vi "Camera_Config.vi"(5 "Crop?":bool, 6 "Camera":T5, 7 "error in":errorcluster, 8 "input cluster":T1={"L16 Linear Actuator"="", "XE 1000 Pump"="", "Camera1"="", "Camera2"="", "Camera1_IMG"=refnum, "Camera2_IMG"=refnum, "Img_Capt"=FALSE, "Actuator"=FALSE, "Pump"=FALSE, "Cam 1"=FALSE, "Cam 2"=FALSE, "Empty_Refill"=FALSE, "Crop"=FALSE, "Light intensity"=100, "Exposure Time"=1000.0, "Sample Name"="Test Sample", "Operator"="MRJ", "Calibration 1"=path "C:/Users/au540322/Desktop/IHS_Project/images/Debris/Debris_0/Debris_0_2019_06_01-23-32-49-686.PNG", "Calibration 2"=path "C:/Users/au540322/Desktop/IHS_Project/images/Debris/Debris_0/Debris_0_2019_06_01-23-32-49-686.PNG", "Framerate"=1, "Timeout Sample"=0, "Collection date"="MRJ", "Sample size threshold"=1, "Empty start"=1, "Command"="MRJ", "Calibration Image 1"=refnum, "Calibration Image 2"=refnum, "Original Image 1"=refnum, "Original Image 2"=refnum, "Processing Image 1"=refnum, "Processing Image 2"=refnum, "Object Image 1"=refnum, "Object Image 2"=refnum, "Cam 1 - save queue"=refnum, "Cam 2 - save queue"=refnum, "Station"="", "Species Name"="", "Other Notes"="", "Aperture"=enum."Item 0", "Image Process Queue Size"=500, "Image Save Queue Size"=500, "Overload threshold"=500, "Max Framerate"=100, "Blue Plane Image"=refnum, "Subtract Image"=refnum, "Binary Image 1"=refnum, "ROI mask allocation"=refnum, "Rectangle 1"={"Left"=0, "Top"=0, "Right"=0, "Bottom"=0, "Rotation"=0.0}, "Rectangle 2"={"Left"=0, "Top"=0, "Right"=0, "Bottom"=0, "Rotation"=0.0}, "Binary Image 2"=refnum, "Detection Region %"=0.0, "Cam 1 queue"=refnum, "Cam 2 queue"=refnum, "Detect image 1"=refnum, "Detect image 2"=refnum, "Detect 1"=path "C:/Users/au540322/Desktop/IHS_Project/images/Debris/Debris_0/Debris_0_2019_06_01-23-32-49-686.PNG", "Detect 2"=path "C:/Users/au540322/Desktop/IHS_Project/images/Debris/Debris_0/Debris_0_2019_06_01-23-32-49-686.PNG", "Max large object threshold"=0, "Open(T)/Close(F)"=FALSE} {"Rectangle 2"."Rotation" format="%.2f"; "Rectangle 2"."Left" scale=0.0..1024.0; "Rectangle 2"."Right" scale=0.0..1024.0; "Rectangle 1"."Rotation" format="%.2f"; "Rectangle 1"."Left" scale=0.0..1024.0; "Rectangle 1"."Right" scale=0.0..1024.0; "Max Framerate" min=1; "Overload threshold" min=1; "Image Save Queue Size" min=1; "Image Process Queue Size" min=1; "Empty start" min=1; "Sample size threshold" min=1; "Framerate" min=1; "Light intensity" scale=0.0..100.0}, 9 "Detect Movement":bool, 10 "Refnum in":T2="cam2") -> (0 "error out":errorcluster, 3 "Refnum out":T2="cam2")   [LabVIEW 2019]
doc: "Configures basler cameras for image acquisition with cropped aspectratio."
uses:
  <vilib>/userdefined/High Color/IMAQdx.ctl
  Camera_ID.ctl
  controls/Data.ctl
  <vilib>/vision/Image Controls.llb/IMAQ Image.ctl
  <resource>/objmgr/imaqdx.rc
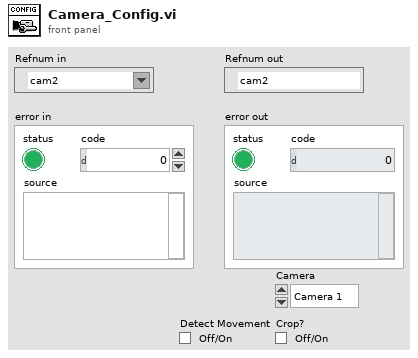
[diagram p1: front panel]
types:
  T1 = typedef "Data.ctl" = cluster{"L16 Linear Actuator":refnum<visa-resource-name>, "XE 1000 Pump":refnum<visa-resource-name>, "Camera1":T2, "Camera2":T2, "Camera1_IMG":T3, "Camera2_IMG":T3, "Img_Capt":bool, "Actuator":bool, "Pump":bool, "Cam 1":bool, "Cam 2":bool, "Empty_Refill":bool, "Crop":bool, "Light intensity":i32, "Exposure Time":dbl, "Sample Name":string, "Operator":string, "Calibration 1":path, "Calibration 2":path, "Framerate":i32, "Timeout Sample":i32, "Collection date":string, "Sample size threshold":i32, "Empty start":u32, "Command":string, "Calibration Image 1":T3, "Calibration Image 2":T3, "Original Image 1":T3, "Original Image 2":T3, "Processing Image 1":T3, "Processing Image 2":T3, "Object Image 1":T3, "Object Image 2":T3, "Cam 1 - save queue":refnum<queue>, "Cam 2 - save queue":refnum<queue>, "Station":string, "Species Name":string, "Other Notes":string, "Aperture":enum32{"Item 0", "Item 1", "Item 2", "Item 3"}, "Image Process Queue Size":i32, "Image Save Queue Size":i32, "Overload threshold":i32, "Max Framerate":i32, "Blue Plane Image":T3, "Subtract Image":T3, "Binary Image 1":T3, "ROI mask allocation":T3, "Rectangle 1":T4, "Rectangle 2":T4, "Binary Image 2":T3, "Detection Region %":dbl, "Cam 1 queue":refnum<queue>, "Cam 2 queue":refnum<queue>, "Detect image 1":T3, "Detect image 2":T3, "Detect 1":path, "Detect 2":path, "Max large object threshold":i32, "Open(T)/Close(F)":bool}
  T2 = typedef "IMAQdx.ctl" = refnum<k21>
  T3 = typedef "IMAQ Image.ctl" = refnum<image>
  T4 = typedef "IMAQ Rectangle" = cluster{"Left":i32, "Top":i32, "Right":i32, "Bottom":i32, "Rotation":dbl}
  T5 = typedef "Camera_ID.ctl" = enum16{"Camera 1", "Camera 2"}
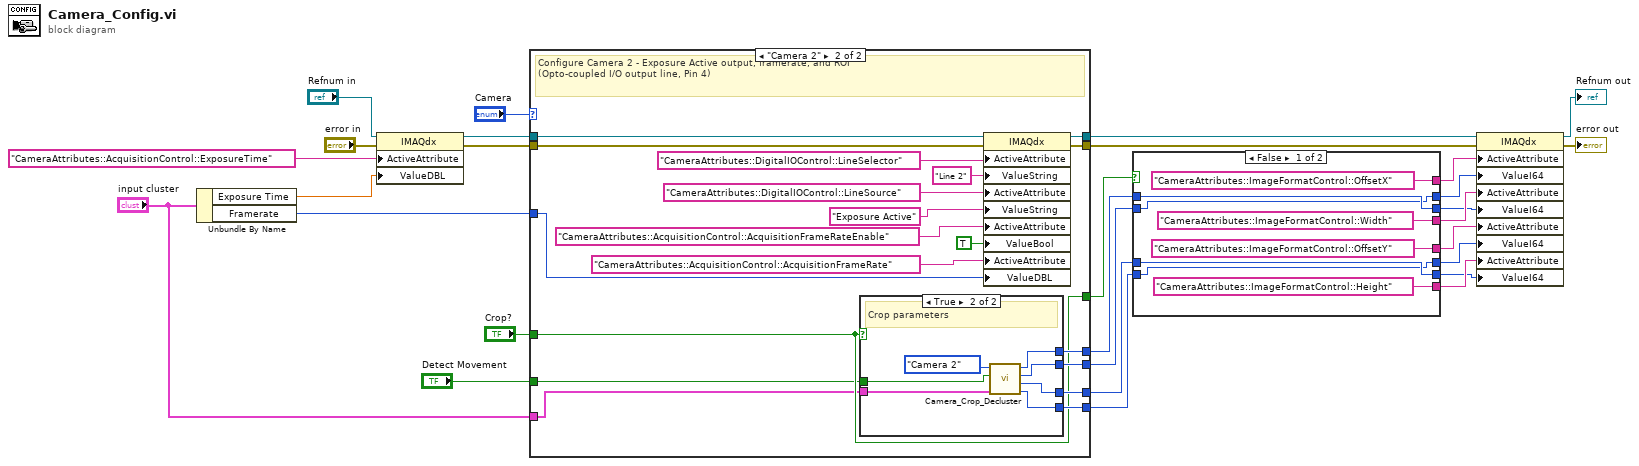
[diagram p0: block diagram]
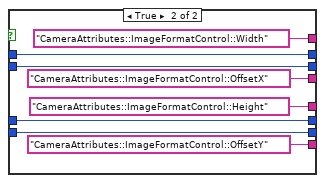
[diagram p2: hidden frame]
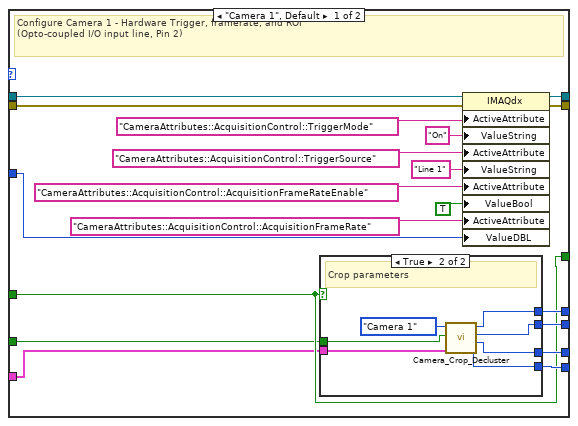
[diagram p3: hidden frame]
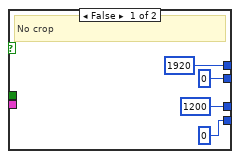
[diagram p4: hidden frame]
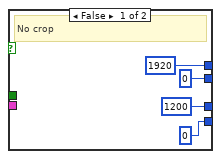
[diagram p5: hidden frame]
diagram:
  n1 = Unbundle By Name("input cluster") -> ("Exposure Time"=w23:dbl, "Framerate"=w22:i32)
  n2 = property class="IMAQdx"(reference="Refnum in", error in="error in", "ActiveAttribute"="CameraAttributes::AcquisitionControl::ExposureTime", "ValueDBL"=w23) -> (reference out=w14:T2, error out=w25:errorcluster)
  n3 = case shown="\"Camera 2\"" "Camera" {
    tunnel: w14 -> [w47 w76]
    tunnel: [w46 w74] -> w12
    tunnel: w25 -> [w45 w75]
    tunnel: [w44 w73] -> w21
    tunnel: w22 -> [w36 w66]
    tunnel: [w34 w65] -> w6
    tunnel: [w35 w64] -> w9
    tunnel: [w32 w62] -> w4
    tunnel: [w33 w63] -> w8
    tunnel: "Crop?" -> [w31 w61]
    tunnel: [w31 w61] -> w11
    tunnel: "input cluster" -> [w30 w60]
    tunnel: "Detect Movement" -> [w29 w59]
    frame "Camera 1", Default {
      # "Configure Camera 1 - Hardware Trigger, framerate, and ROI \n(Opto-coupled I/O input line, Pin 2)"
      n4 = case shown="True" w31 {
        tunnel: [i64 1920 w57] -> w35
        tunnel: [1200 w55] -> w34
        tunnel: [i64 0 w56] -> w33
        tunnel: [0 w54] -> w32
        tunnel: w30 -> [_ w53]
        tunnel: w29 -> [_ w52]
        frame False {
          # "No crop"
        }
        frame True {
          # "Crop parameters"
          n5 = call "Camera_Crop_Decluster.vi"("input cluster"=w53, "Detect Movement"=w52, "Camera"=Camera_ID."Camera 1") -> ("OffsetY"=w54:i64, "Height"=w55:i64, "OffsetX"=w56:i64, "Width"=w57:i64)  [unwired: 5 in]
        }
      }
      n6 = property class="IMAQdx"(reference=w47, error in=w45, "ActiveAttribute"="CameraAttributes::AcquisitionControl::TriggerMode", "ValueString"="On", "ActiveAttribute"="CameraAttributes::AcquisitionControl::TriggerSource", "ValueString"="Line 1", "ActiveAttribute"="CameraAttributes::AcquisitionControl::AcquisitionFrameRateEnable", "ValueBool"=TRUE, "ActiveAttribute"="CameraAttributes::AcquisitionControl::AcquisitionFrameRate", "ValueDBL"=w36) -> (reference out=w46:T2, error out=w44:errorcluster)
    }
    frame "Camera 2" {
      # "Configure Camera 2 - Exposure Active output, framerate, and ROI\n(Opto-coupled I/O output line, Pin 4)"
      n7 = case shown="True" w61 {
        tunnel: [1200 w84] -> w65
        tunnel: [i64 1920 w86] -> w64
        tunnel: [i64 0 w85] -> w63
        tunnel: [0 w83] -> w62
        tunnel: w60 -> [_ w88]
        tunnel: w59 -> [_ w82]
        frame False {
          # "No crop"
        }
        frame True {
          # "Crop parameters"
          n8 = call "Camera_Crop_Decluster.vi"("input cluster"=w88, "Detect Movement"=w82, "Camera"=Camera_ID."Camera 2") -> ("OffsetY"=w83:i64, "Height"=w84:i64, "OffsetX"=w85:i64, "Width"=w86:i64)  [unwired: 5 in]
        }
      }
      n9 = property class="IMAQdx"(reference=w76, error in=w75, "ActiveAttribute"="CameraAttributes::DigitalIOControl::LineSelector", "ValueString"="Line 2", "ActiveAttribute"="CameraAttributes::DigitalIOControl::LineSource", "ValueString"="Exposure Active", "ActiveAttribute"="CameraAttributes::AcquisitionControl::AcquisitionFrameRateEnable", "ValueBool"=TRUE, "ActiveAttribute"="CameraAttributes::AcquisitionControl::AcquisitionFrameRate", "ValueDBL"=w66) -> (reference out=w74:T2, error out=w73:errorcluster)
    }
  }
  n10 = case shown="False" w11 {
    tunnel: ["CameraAttributes::ImageFormatControl::Height" ("ActiveAttribute") "CameraAttributes::ImageFormatControl::OffsetY" ("ActiveAttribute")] -> w20
    tunnel: ["CameraAttributes::ImageFormatControl::OffsetY" ("ActiveAttribute") "CameraAttributes::ImageFormatControl::Height" ("ActiveAttribute")] -> w19
    tunnel: ["CameraAttributes::ImageFormatControl::Width" ("ActiveAttribute") "CameraAttributes::ImageFormatControl::OffsetX" ("ActiveAttribute")] -> w18
    tunnel: ["CameraAttributes::ImageFormatControl::OffsetX" ("ActiveAttribute") "CameraAttributes::ImageFormatControl::Width" ("ActiveAttribute")] -> w17
    tunnel: [w91 w100] -> w10
    tunnel: w9 -> [w92 w100]
    tunnel: w8 -> [w91 w99]
    tunnel: [w92 w99] -> w7
    tunnel: w6 -> [w90 w98]
    tunnel: [w89 w98] -> w5
    tunnel: w4 -> [w89 w97]
    tunnel: [w90 w97] -> w3
    frame False {
    }
    frame True {
    }
  }
  n11 = property class="IMAQdx"(reference=w12, error in=w21, "ActiveAttribute"=w17, "ValueI64"=w10, "ActiveAttribute"=w18, "ValueI64"=w7, "ActiveAttribute"=w19, "ValueI64"=w5, "ActiveAttribute"=w20, "ValueI64"=w3) -> (reference out=→"Refnum out":T2, error out=→"error out":errorcluster)
